vi "Query Setpoint.vi"(0 "VISA resource name":refnum<visa-resource-name>, 11 "error in (no error)":errorcluster) -> (4 "VISA resource name out":refnum<visa-resource-name>, 6 "Voltage Setpoint (volts)":dbl, 8 "Current Setpoint (amps)":dbl, 10 "Power Setpoint (watts)":dbl, 15 "error out":errorcluster)   [LabVIEW 2018, in "XP Power PLS600.lvlib"]
doc: "Queries the present voltage, current, and power setpoints."
uses:
  XP Power PLS600.lvlib
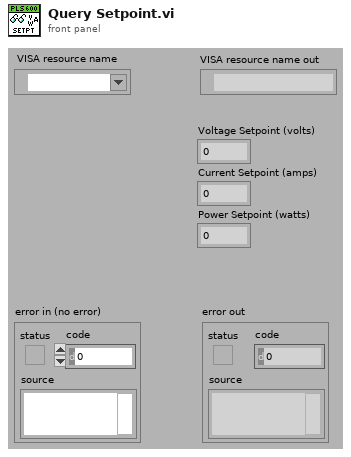
[diagram p1: front panel]
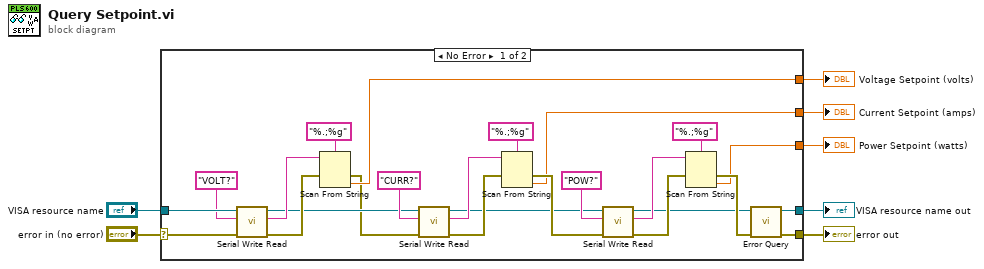
[diagram p0: block diagram]
diagram:
  n1 = case shown="No Error" "error in (no error)" {
    selector: "error in (no error)" -> [w24 w34]
    tunnel: [w32 w33] -> w7
    tunnel: [w31 w34] -> w6
    tunnel: [w29 _] -> w5
    tunnel: "VISA resource name" -> [w28 w33]
    tunnel: [w9 _] -> w2
    tunnel: [w8 _] -> w1
    frame No Error {
      n2 = call "Serial Write Read.vi"("error in (no error)"=w24, "Write Buffer"="VOLT?", "VISA resource name"=w28) -> ("error out"=w25:errorcluster, "Read Buffer"=w26:string, "VISA resource name out"=w15:refnum<visa-resource-name>)  [unwired: 6 in]
      n3 = Scan From String(format string="%.;%g", input string=w26, error in=w25) -> (error out=w14:errorcluster, output 1=w29:dbl)  [unwired: 2 in, 2 out]
      n4 = call "Serial Write Read.vi"("error in (no error)"=w14, "Write Buffer"="CURR?", "VISA resource name"=w15) -> ("error out"=w20:errorcluster, "Read Buffer"=w21:string, "VISA resource name out"=w12:refnum<visa-resource-name>)  [unwired: 6 in]
      n5 = Scan From String(format string="%.;%g", input string=w21, error in=w20) -> (error out=w13:errorcluster, output 1=w9:dbl)  [unwired: 2 in, 2 out]
      n6 = call "Serial Write Read.vi"("error in (no error)"=w13, "Write Buffer"="POW?", "VISA resource name"=w12) -> ("error out"=w16:errorcluster, "Read Buffer"=w17:string, "VISA resource name out"=w10:refnum<visa-resource-name>)  [unwired: 6 in]
      n7 = Scan From String(format string="%.;%g", input string=w17, error in=w16) -> (error out=w11:errorcluster, output 1=w8:dbl)  [unwired: 2 in, 2 out]
      n8 = call "Error Query.vi"("error in (no error)"=w11, "VISA resource name"=w10) -> ("error out"=w31:errorcluster, "VISA resource name out"=w32:refnum<visa-resource-name>)  [unwired: 6 in, 2 out]
    }
    frame Error {
    }
  }
  "VISA resource name out" <- w7
  "error out" <- w6
  "Voltage Setpoint (volts)" <- w5
  "Power Setpoint (watts)" <- w1
  "Current Setpoint (amps)" <- w2
